vi "Fish Census.vi"() -> ()   [LabVIEW 2020]
uses:
  <vilib>/regexp/Match Regular Expression.xnode
panel:
  in  "# Days":i32=256
  out "Total":i64
  in  "Input":string="3,1,4,2,1,1,1,1,1,1,1,4,1,4,1,2,1,1,2,1,3,4,5,1,1,4,1,3,3,1,1,1,1,3,3,1,3,3,1,5,5,1,1,3,1,1,2,1,1,1,3,1,4,3,2,1,4,3,3,1,1,1,1,5,1,4,1,1,1,4,1,4,4,1,5,1,1,4,5,1,1,2,1,1,1,4,1,2,1,1,1,1,1,1,5,1,3,1,1,4,4,1,1,5,1,2,1,1,1,1,5,1,3,1,1,1,2,2,1,4,1,3,1,4,1,2,1,1,1,1,1,3,2,5,4,4,1,3,2,1,4,1,3,1,1,1,2,1,1,5,1,2,1,1,1,2,1,4,3,1,1,1,4,1,1,1,1,1,2,2,1,1,5,1,1,3,1,2,5,5,1,4,1,1,1,1,1,2,1,1,1,1,4,5,1,1,1,1,1,1,1,1,1,3,4,4,1,1,4,1,3,4,1,5,4,2,5,1,2,1,1,1,1,1,1,4,3,2,1,1,3,2,5,2,5,5,1,3,1,2,1,1,1,1,1,1,1,1,1,3,1,1,1,3,1,4,1,4,2,1,3,4,1,1,1,2,3,1,1,1,4,1,2,5,1,2,1,5,1,1,2,1,2,1,1,1,1,4,3,4,1,5,5,4,1,1,5,2,1,3"
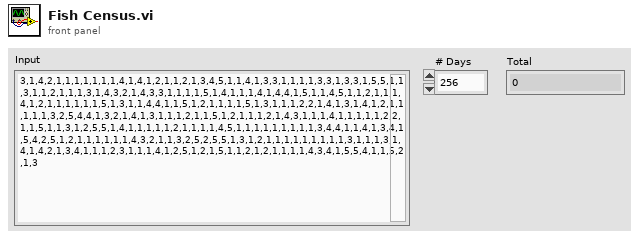
[diagram p1: front panel]
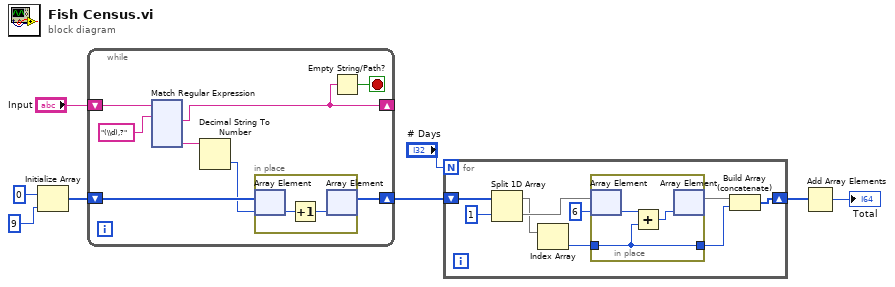
[diagram p0: block diagram]
diagram:
  n1 = Initialize Array(i64 0, 9 ("dimension size")) -> (w5:i64[])
  n2 = while {
    shift-right: [w13] -> _
    shift-left: "Input" -> [w16]
    shift-right: [w9] -> w4
    shift-left: w5 -> [w11]
    stop <- w14 stop-if-true
    n3 = xnode "Match Regular Expression"("input string"=w16, "regular expression"="(\\d),?") -> ("after match"=w13:string, "submatch 1"=w12:string)  [unwired: 4 in, 4 out]
    n4 = Decimal String To Number(string=w12) -> (number=w10:i32)  [unwired: 2 in, 1 out]
    n5 = in-place {
      n6 = in-place-array #1(w11, w10) -> (w18:i64)
      n7 = Increment(x=w18) -> (x+1=w17:i64)
      n8 = in-place-array #1(w17) -> (w9:i64[])  [unwired: 1 out]
    }
    n9 = Empty String/Path?(string/path=w13) -> (empty?=w14:bool)
  }
  n10 = for {
    N: "# Days" -> [_]
    shift-right: [w135] -> w2
    shift-left: w4 -> [w142]
    n11 = Split 1D Array(array=w142, index=1 ("length")) -> (first subarray=w139:i64[], second subarray=w140:i64[])
    n12 = Index Array(array=w139) -> (element=w138:i64)  [unwired: 1 in]
    n13 = in-place {
      in-place-border: w138 -> [w144]
      in-place-border: [w144] -> w136
      n14 = in-place-array #2(w140, 6) -> (w146:i64)
      n15 = Add(x=w146, y=w144) -> (x+y=w145:i64)
      n16 = in-place-array #2(w145) -> (w137:i64[])  [unwired: 1 out]
    }
    n17 = Build Array (concatenate)(w137, w136) -> (w135:i64[])
  }
  n18 = Add Array Elements(numeric array=w2) -> (sum=→"Total":i64)
